vi "daqio_Delete_File.vi"(8 "error in (no error)":errorcluster, 10 "daq.io file ID":string, 11 "daq.io type in":T1={"daq.io ref"=refnum, "daq.io API Base"="http://dashboard.daq.io/api/v1", "Device Type Key"="", "Device Key"="", "Account ID"="", "online"=TRUE, "SSL"=TRUE}) -> (0 "error out":errorcluster, 3 "daq.io type out":T1={"daq.io ref"=refnum, "daq.io API Base"="http://dashboard.daq.io/api/v1", "Device Type Key"="", "Device Key"="", "Account ID"="", "online"=TRUE, "SSL"=TRUE})   [LabVIEW 2013, in "daqio minimal.lvlib"]
doc: "This VI deletes a specified user file. Please specifiy the file to delete by its unique file ID. To retrieve the file IDs you can use the \"Get all Files\" function and search its output array."
uses:
  daqio minimal.lvlib
  _typedefs/daqio-Type.ctl
  <vilib>/httpClient/ClientHandle.ctl
  <vilib>/Easy HTTP Client/Easy HTTP.lvlib
  <vilib>/httpClient/LabVIEWHTTPClient.lvlib
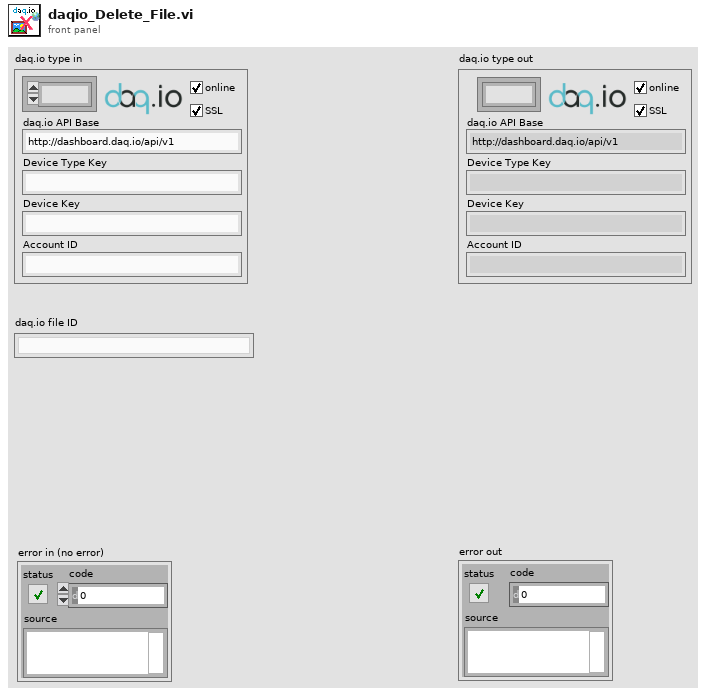
[diagram p1: front panel]
types:
  T1 = typedef "daqio minimal.lvlib/daqio-Type.ctl" = cluster{"daq.io ref":T2, "daq.io API Base":string, "Device Type Key":string, "Device Key":string, "Account ID":string, "online":bool, "SSL":bool}
  T2 = typedef "LabVIEWHTTPClient.lvlib/ClientHandle.ctl" = refnum<k1>
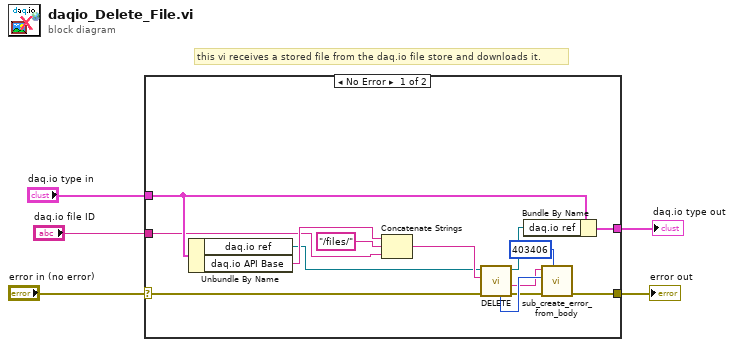
[diagram p0: block diagram]
diagram:
  # "this vi receives a stored file from the daq.io file store and downloads it."
  n1 = case shown="No Error" "error in (no error)" {
    selector: "error in (no error)" -> [w7 w20]
    tunnel: "daq.io type in" -> [w16 w21]
    tunnel: [w15 w21] -> w4
    tunnel: [w18 w20] -> w3
    tunnel: "daq.io file ID" -> [w11 _]
    frame No Error {
      n2 = Unbundle By Name(w16) -> ("daq.io ref"=w6:T2, "daq.io API Base"=w17:string)
      n3 = Concatenate Strings(w17, "/files/", w11) -> (w8:string)
      n4 = call <vilib>:"DELETE.vi"("error in (no error)"=w7, "url"=w8, "client handle"=w6) -> ("error out"=w12:errorcluster, "body"=w9:string, "client handle out"=w13:T2, "HTTP Response Code"=w14:i32)  [unwired: 4 in, 1 out]
      n5 = Bundle By Name(cluster=w16, "daq.io ref"=w13) -> (w15:T1)
      n6 = call "sub_create_error_from_body.vi"("error code"=403406, "error in (no error)"=w12, "http code"=w14, "body"=w9) -> ("error out"=w18:errorcluster)  [unwired: 7 in]
    }
    frame Error {
    }
  }
  "error out" <- w3
  "daq.io type out" <- w4
